vi "Bootstrapping Password.vi"(0 "User Manager Model in":refnum<class "User Manager Model.lvclass">) -> (4 "User Manager Model out":refnum<class "User Manager Model.lvclass">, 6 "Username":string, 8 "Password":string, 10 "User Level":T1, 15 "User Levels In This Society":T1[](array[typedef]))   [LabVIEW 2020, in "User Manager Model.lvlib" / "User Manager Model.lvclass"]
uses:
  <vilib>/gpm_packages/@cs/User Manager App/User Manager Model/User Manager Model/User Manager Model.lvclass
  <vilib>/gpm_packages/@cs/User Manager App/User Manager Model/Type Definitions/User Levels.ctl
  <vilib>/gpm_packages/@cs/User Manager App/User Manager Model/User Manager Model/User Manager Model.lvclass/User Manager Model.ctl
  <vilib>/gpm_packages/@cs/User Manager App/User Manager Model/Type Definitions/User Manager Application Types.lvlib
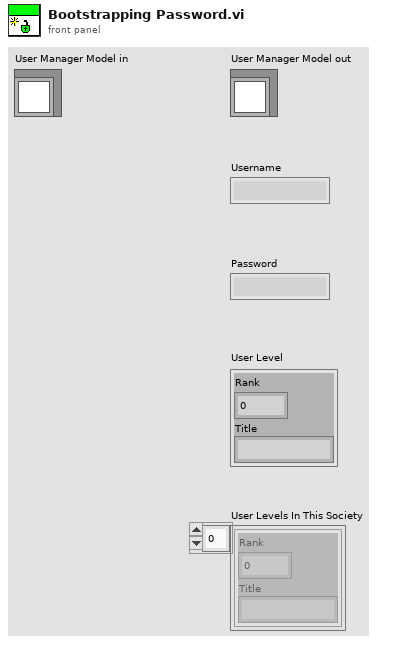
[diagram p1: front panel]
types:
  T1 = typedef "User Manager Application Types.lvlib/User Levels.ctl" = cluster{"Rank":i32, "Title":string}
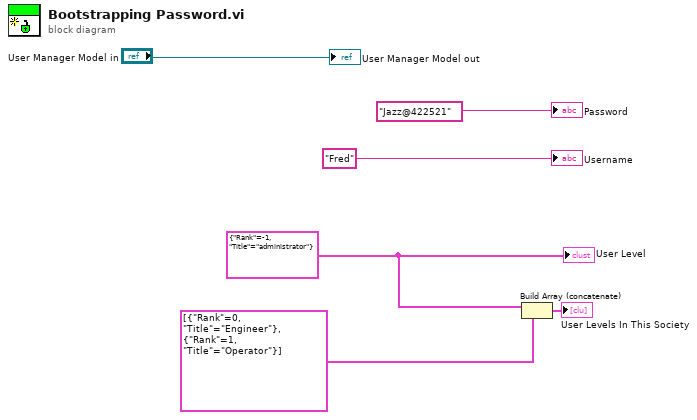
[diagram p0: block diagram]
diagram:
  w5 = T1 {"Rank"=-1, "Title"="administrator"} ("User Level")
  n1 = Build Array (concatenate)(w5, T1[] [{"Rank"=0, "Title"="Engineer"}, {"Rank"=1, "Title"="Operator"}]) -> (→"User Levels In This Society":T1[])
  "User Manager Model out" <- "User Manager Model in"
  "Username" <- "Fred"
  "Password" <- "Jazz@422521"
  "User Level" <- w5
